vi "Is Safe to Destroy Refnums.vi"(8 "error in (no error)":errorcluster, 11 "Module Admin":refnum<class "Delacor_lib_QMH_Cloneable Module Admin.lvclass">) -> (0 "error out":errorcluster, 3 "Destroy Broadcast & Request Event Refs?":bool)   [LabVIEW 2015, in "Chat Window.lvlib"]
doc: "If this cloneable module instance was the first one that was launched, wait until all other instances are closed, then indicate that it is safe to destroy the event references.\n_____\nBased on Delacor QMH Project Template 4.2.1.64."
uses:
  Chat Window.lvlib
  Clone Registration/Clone Registration.lvlib
  <vilib>/Delacor/Delacor QMH/Libraries/Cloneable Module Admin_class/Delacor_lib_QMH_Cloneable Module Admin.lvclass
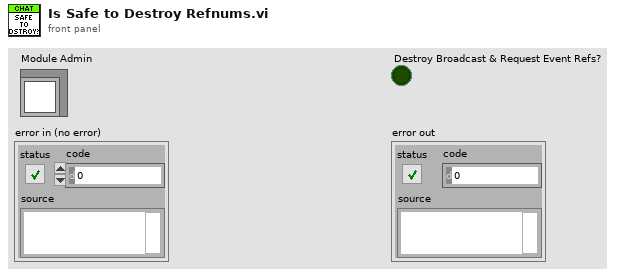
[diagram p1: front panel]
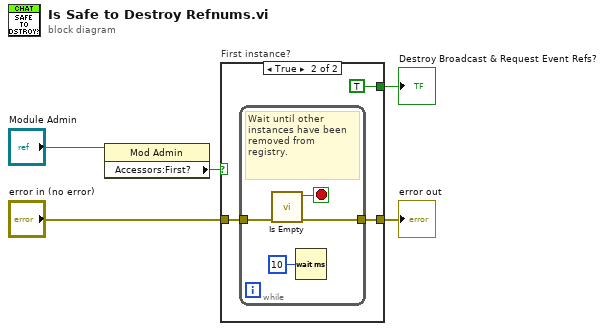
[diagram p0: block diagram]
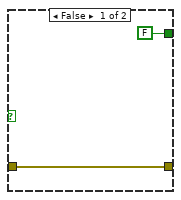
[diagram p2: hidden frame]
diagram:
  n1 = property class="Mod Admin"(reference="Module Admin") -> ("Accessors:First?"=w1:bool)  [unwired: 1 in, 2 out]
  n2 = case "First instance?" shown="True" w1 {
    tunnel: "error in (no error)" -> [w7 w10]
    tunnel: [w7 w9] -> w4
    tunnel: [FALSE TRUE] -> w5
    frame False {
    }
    frame True {
      n3 = while {
        tunnel: w10 -> [w13]
        tunnel: [w12] -> w9
        stop <- w14 stop-if-true
        # "Wait until other instances have been removed from registry."
        n4 = call "Is Empty.vi"("error in (no error)"=w13) -> ("error out"=w12:errorcluster, "Empty?"=w14:bool)  [unwired: 9 in]
        n5 = Wait (ms)(milliseconds to wait=u32 10) -> ()  [unwired: 1 out]
      }
    }
  }
  "Destroy Broadcast & Request Event Refs?" <- w5
  "error out" <- w4
